vi "test_TxGen-RxMon_Redundant.vi"(8 "error in":errorcluster, 11 "reference in":refnum<class "AIM ARINC 664 Loopback.lvclass">) -> (0 "error out":errorcluster, 3 "reference out":refnum<class "AIM ARINC 664 Loopback.lvclass">)   [LabVIEW 2020, in "AIM ARINC 664 Loopback.lvclass"]
uses:
  AIM ARINC 664 Loopback.lvclass
  AIM ARINC 664 Loopback.lvclass/AIM ARINC 664 Loopback.ctl
  <vilib>/addons/_JKI Toolkits/VI Tester/TestCase.llb/TestCase.lvclass
  NationalInstruments.VeriStand.SystemDefinitionAPI
  b47c41b5-a02e-49d5-b852-4e28f097d7ad.vi
  Scripting/AIM ARINC 664 Scripting.lvlib
  <vilib>/NI VeriStand/Execution/Workspace/NI_VS Workspace ExecutionAPI.lvlib
  73f22a09-5042-4cee-9c03-739189b9d92e.vi
  98b0eca8-d5c5-4990-8264-b33462e0ad74.vi
  <vilib>/NI VeriStand/Execution/Workspace/NI VeriStand - Get Multiple Channel Values.vi
  <vilib>/NI VeriStand/Custom Device API/Custom Device API.lvlib
  C:/Program Files/National Instruments/LabVIEW 2025/vi.lib/addons/_JKI Toolkits/VI Tester/TestCase.llb/TestCase.lvclass
panel:
  in  "Time Target (s)":dbl=5.0
  in  "tolerance (5 samples)":dbl=20.0 caption="Time Target (s)"
  out "Values":dbl[](array[numeric])
  out "Elapsed Time (s)":dbl
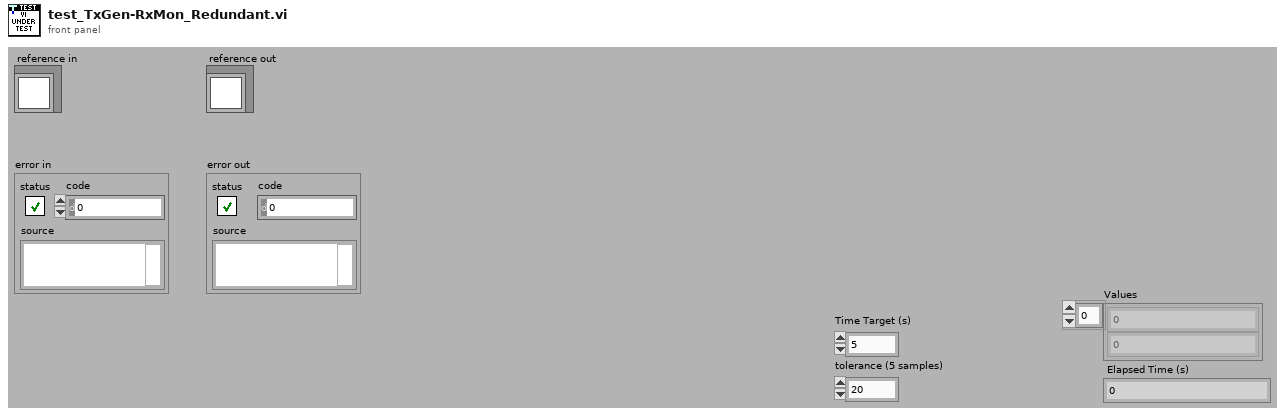
[diagram p1: front panel]
types:
  T1 = typedef "Custom Device API.lvlib/Custom Device Item Ref.ctl" = u64
  T2 = typedef "Custom Device API.lvlib/Custom Device Item Info.ctl" = cluster{"Name":string, "Is Channel":bool, "GUID":string, "Is Waveform":bool}
  T3 = typedef "NI_VS Workspace ExecutionAPI.lvlib/WorkspaceAPI.ctl" = refnum<k24>
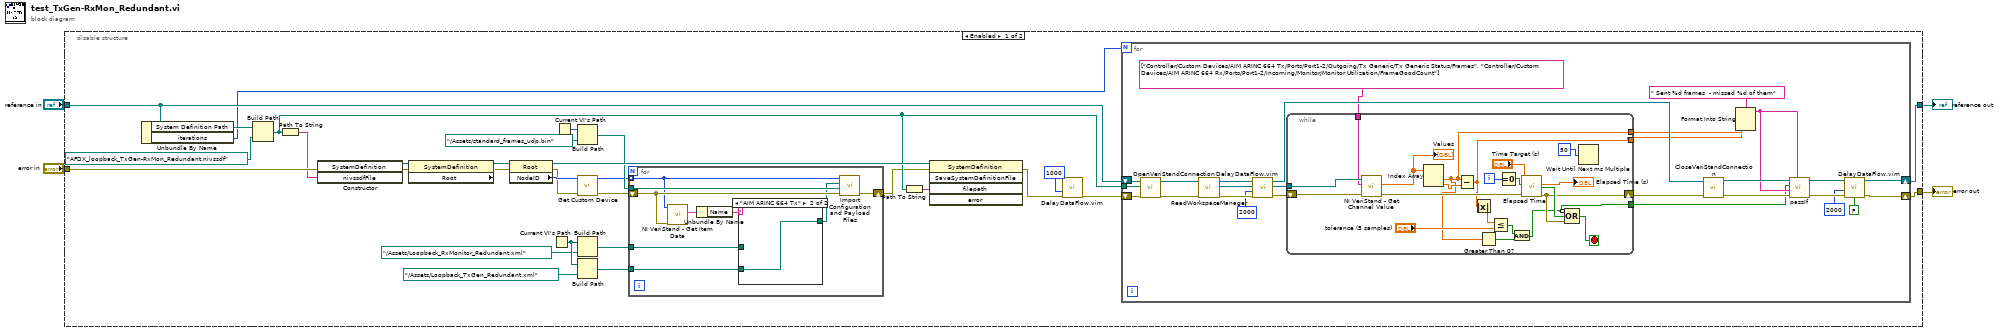
[diagram p0: block diagram]
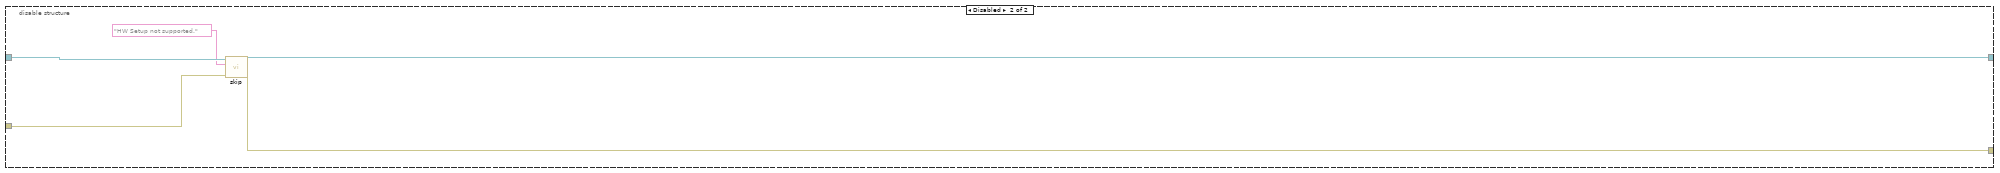
[diagram p3: hidden frame]
diagram:
  n1 = disable-structure shown="Enabled" {
    disable-tunnel: "reference in" -> [w17 w96]
    disable-tunnel: "error in" -> [w33 w95]
    disable-tunnel: [w13 w94] -> w2
    disable-tunnel: [w14 w93] -> w1
    frame Enabled {
      n2 = Unbundle By Name(w17) -> ("System Definition Path"=w35:path, "iterations"=w15:i32)
      n3 = Build Path(base path=w35, name or relative path=path "AFDX_loopback_TxGen-RxMon_Redundant.nivssdf") -> (appended path=w16:path)
      n4 = Path To String(path=w16) -> (string=w32:string)
      n5 = constructor class="SystemDefinition"(error in=w33, "nivssdfFile"=w32) -> (reference out=w31:refnum<k24>, error out=w29:errorcluster)  [unwired: 2 in, 2 out]
      n6 = property class="SystemDefinition"(reference=w31, error in=w29) -> (reference out=w25:refnum<k24>, error out=w28:errorcluster, "Root"=w30:refnum<k24>)
      n7 = property class="Root"(reference=w30, error in=w28) -> (error out=w22:errorcluster, "NodeID"=w23:u64)  [unwired: 1 out]
      n8 = Current VI's Path() -> (path=w19:path)
      n9 = Current VI's Path() -> (path=w27:path)
      n10 = Build Path(base path=w27, name or relative path=path "../Assets/standard_frames_udp.bin") -> (appended path=w8:path)
      n11 = call "Get Custom Device.vi"("error in"=w22, "custom device ref in"=w23) -> ("error out"=w6:errorcluster, "Item Refs"=w7:T1[])  [unwired: 5 in, 3 out]
      n12 = Build Path(base path=w19, name or relative path=path "../Assets/Loopback_RxMonitor_Redundant.xml") -> (appended path=w10:path)
      n13 = Build Path(base path=w19, name or relative path=path "../Assets/Loopback_TxGen_Redundant.xml") -> (appended path=w9:path)
      n14 = for {
        tunnel: w8 -> [w44]
        tunnel: w7 -> [w37] mode=indexing
        shift-right: [w43] -> w5
        shift-left: w6 -> [w42]
        tunnel: w9 -> [w38]
        tunnel: w10 -> [w36]
        n15 = call <vilib>:"NI VeriStand - Get Item Data.vi"("error in (no error)"=w42, "Item Ref in"=w37) -> ("Item Info"=w41:T2)  [unwired: 6 in, 3 out]
        n16 = Unbundle By Name(w41) -> ("Name"=w40:string)
        n17 = case shown="\"AIM ARINC 664 Tx\"" w40 {
          tunnel: [w45 w46] -> w39
          tunnel: w38 -> [_ w46]
          tunnel: w36 -> [w45 _]
          frame "AIM ARINC 664 Rx", Default {
          }
          frame "AIM ARINC 664 Tx" {
          }
        }
        n18 = call "Import Configuration and Payload Files.vi"("error in"=w42, "payload file path"=w44, "parameters configuration file path"=w39, "custom device ref"=w37) -> ("error out"=w43:errorcluster)  [unwired: 6 in, 1 out]
      }
      n19 = Path To String(path=w16) -> (string=w24:string)
      n20 = invoke class="SystemDefinition" method="SaveSystemDefinitionFile"(reference=w25, error in=w5, "filepath"=w24) -> (error out=w21:errorcluster)  [unwired: 2 in, 4 out]
      n21 = call "DelayDataFlow.vim"("value in"=w21, "milliseconds to wait"=u32 1000) -> ("value out"=w18:errorcluster)  [unwired: 2 in, 1 out]
      n22 = for {
        N: w15 -> [_]
        tunnel: w16 -> [w52]
        shift-right: [w69] -> w14
        shift-left: w17 -> [w70]
        shift-right: [w50] -> w13
        shift-left: w18 -> [w53]
        n23 = call-dynamic "OpenVeriStandConnection.vi"("error in (no error)"=w53, "System Definition File"=w52, "VeriStand Test Case in"=w70) -> ("error out"=w68:errorcluster, "VeriStand Test Case out"=w63:refnum<class "AIM ARINC 664 Loopback.lvclass">)  [unwired: 6 in, 1 out]
        n24 = call-dynamic "ReadWorkspaceManager.vi"("error in (no error)"=w68, "VeriStand Test Case in"=w63) -> ("error out"=w58:errorcluster, "Workspace"=w61:T3, "VeriStand Test Case out"=w62:refnum<class "AIM ARINC 664 Loopback.lvclass">)  [unwired: 7 in]
        n25 = call "DelayDataFlow.vim"("value in"=w58, "milliseconds to wait"=u32 2000) -> ("value out"=w57:errorcluster)  [unwired: 2 in, 1 out]
        n26 = while {
          tunnel: w61 -> [w91]
          shift-right: [w84] -> w60
          shift-left: w57 -> [w89]
          tunnel: [w77] -> w59
          tunnel: [w76] -> w55
          tunnel: [w75] -> w54
          tunnel: string[] ["Controller/Custom Devices/AIM ARINC 664 Tx/Ports/Port1-2/Outgoing/Tx Generic/Tx Generic Status/Frames", "Controller/Custom Devices/AIM ARINC 664 Rx/Ports/Port1-2/Incoming/Monitor/Monitor Utilization/FrameGoodCount"] ("Channels") -> [w73]
          i -> [w72]
          stop <- w86 stop-if-true
          n27 = call-poly <vilib>:"NI VeriStand - Get Channel Value.vi"("error in (no error)"=w89, "Channels"=w73, "WorkspaceManager in"=w91) -> ("error out"=w88:errorcluster, "Values"=w83:dbl[])  [unwired: 6 in, 1 out]
          "Values" <- w83
          n28 = Index Array(array=w83) -> (element #1=w76:dbl, element #2=w82:dbl)  [unwired: 2 in]
          n29 = Subtract(x=w76, y=w82) -> (x-y=w75:dbl)
          n30 = Absolute Value(x=w75) -> (abs(x)=w81:dbl)
          n31 = Greater Than 0?(x=w76) -> (x > 0?=w78:bool)
          n32 = Less Or Equal?(x=w81, y="tolerance (5 samples)") -> (x <= y?=w79:bool)
          n33 = Equal To 0?(x=w72) -> (x = 0?=w71:bool)
          n34 = And(x=w79, y=w78) -> (x .and. y?=w77:bool)
          n35 = call "Elapsed Time"("Time Target (s)"="Time Target (s)", "Reset"=w71, "error in (no error)"=w88) -> ("Elapsed Time (s)"=→"Elapsed Time (s)":dbl, "Time has Elapsed"=w87:bool, "error out"=w84:errorcluster)  [unwired: 9 in, 5 out]
          n36 = Compound Arithmetic op=OR(invert w77, w87, w84) -> (w86:bool)
          n37 = Wait Until Next ms Multiple(millisecond multiple=u32 50 ("millisecond timer value")) -> ()  [unwired: 1 out]
        }
        n38 = call-dynamic "CloseVeriStandConnection.vi"("error in (no error)"=w60, "VeriStand Test Case in"=w62) -> ("error out"=w67:errorcluster, "VeriStand Test Case out"=w66:refnum<class "AIM ARINC 664 Loopback.lvclass">)  [unwired: 8 in]
        n39 = Format Into String(format string=" Sent %d frames  - missed %d of them", w55, w54) -> (resulting string=w64:string)  [unwired: 2 in, 1 out]
        n40 = call-dynamic "passIf.vi"("custom report message (\"\")"=w64, "error in (no error)"=w67, "message (\"\")"=w64, "pass"=w59, "TestCase in"=w66) -> ("error out"=w49:errorcluster, "TestCase out"=w69:refnum<class "AIM ARINC 664 Loopback.lvclass">)  [unwired: 5 in]
        n41 = call "DelayDataFlow.vim"("value in"=w49, "milliseconds to wait"=u32 2000, "no delay on error (T)"=FALSE) -> ("value out"=w50:errorcluster)  [unwired: 1 in, 1 out]
      }
    }
    frame Disabled {
      n42 = call <vilib>:"skip.vi"("error in (no error)"=w95, "skipMessage"="HW Setup not supported.", "TestCase in"=w96) -> ("error out"=w94:errorcluster, "TestCase out"=w93:refnum<class "AIM ARINC 664 Loopback.lvclass">)  [unwired: 7 in]
    }
  }
  "error out" <- w2
  "reference out" <- w1
